vi "Create_Run_Dir.vi"(11 "Run":string) -> (0 "Run exists":bool, 1 "Time exists":bool, 2 "Date exists":bool, 3 "dup path":path)   [LabVIEW 2018]
panel:
  out "time string":string
  out "date string":string
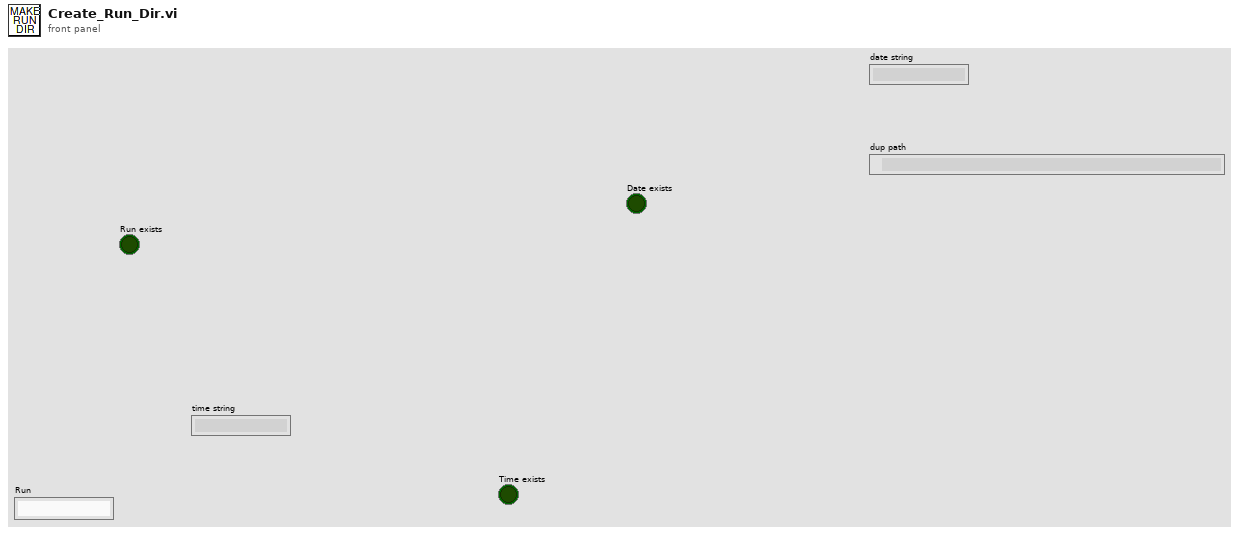
[diagram p1: front panel]
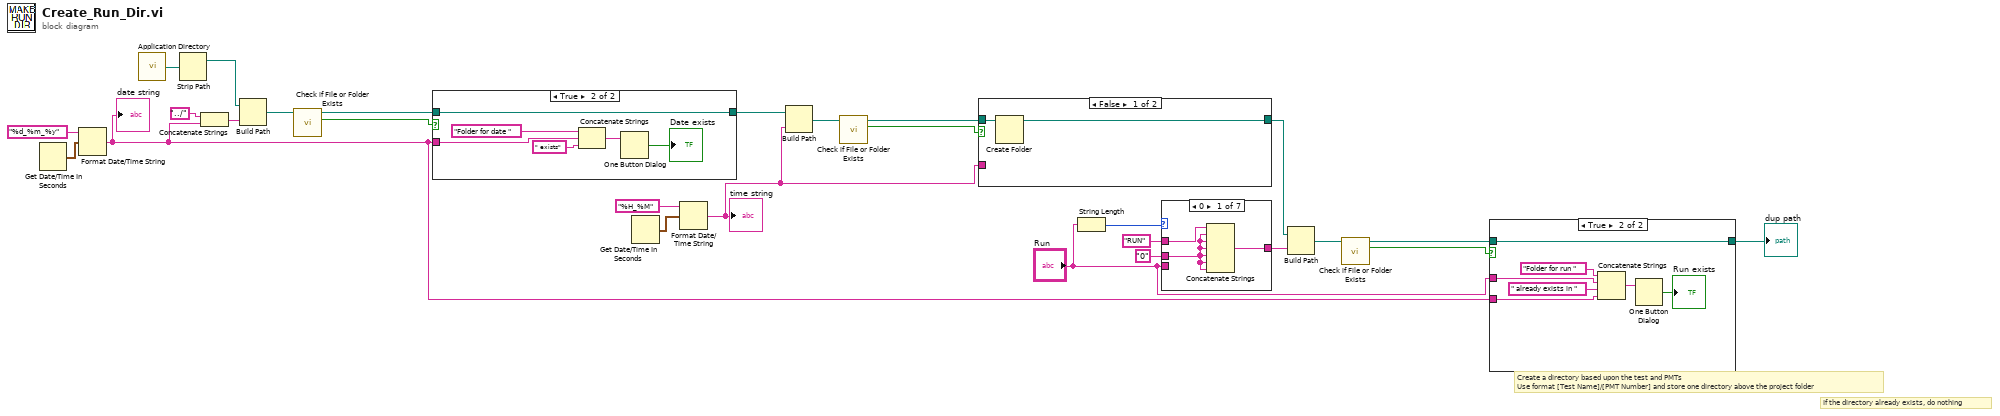
[diagram p0: block diagram]
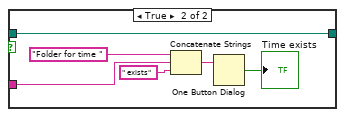
[diagram p2: hidden frame]
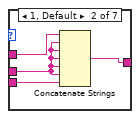
[diagram p3: hidden frame]
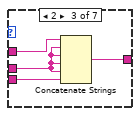
[diagram p4: hidden frame]
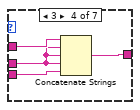
[diagram p5: hidden frame]
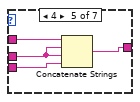
[diagram p6: hidden frame]
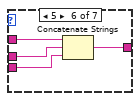
[diagram p7: hidden frame]
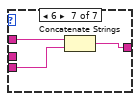
[diagram p8: hidden frame]
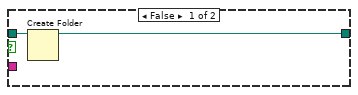
[diagram p9: hidden frame]
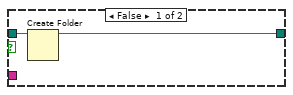
[diagram p10: hidden frame]
diagram:
  # "If the directory already exists, do nothing"
  # "Create a directory based upon the test and PMTs\nUse format [Test Name]/[PMT Number] and store one directory above the project folder"
  n1 = Get Date/Time In Seconds() -> (seconds since 1Jan1904=w22:timestamp)
  n2 = Format Date/Time String(time format string (%c)="%d_%m_%y", seconds (now)=w22) -> (date/time string=w11:string)  [unwired: 1 in]
  "date string" <- w11
  n3 = call <vilib>:"Application Directory.vi"() -> ("Application Directory"=w27:path)
  n4 = Strip Path(path=w27) -> (stripped path=w20:path)  [unwired: 1 out]
  n5 = Concatenate Strings("../" ("string"), w11) -> (w9:string)
  n6 = Build Path(base path=w20, name or relative path=w9) -> (appended path=w18:path)
  n7 = call <vilib>:"Check if File or Folder Exists.vi"("path"=w18) -> ("file or folder exists?"=w19:bool, "dup path"=w17:path)  [unwired: 8 in, 1 out]
  n8 = case shown="True" w19 {
    tunnel: w17 -> [w29 w35]
    tunnel: [w28 w35] -> w3
    tunnel: w11 -> [_ w31]
    frame False {
      n9 = Create Folder(path (use dialog)=w29) -> (created path=w28:path)  [unwired: 2 in, 2 out]
    }
    frame True {
      n10 = Concatenate Strings("Folder for date " ("message"), w31, " exists" ("string")) -> (w33:string)
      n11 = One Button Dialog(message=w33) -> (true=→"Date exists":bool)  [unwired: 1 in]
    }
  }
  n12 = Get Date/Time In Seconds() -> (seconds since 1Jan1904=w8:timestamp)
  n13 = Format Date/Time String(time format string (%c)="%H_%M", seconds (now)=w8) -> (date/time string=w1:string)  [unwired: 1 in]
  "time string" <- w1
  n14 = Build Path(base path=w3, name or relative path=w1) -> (appended path=w2:path)
  n15 = call <vilib>:"Check if File or Folder Exists.vi"("path"=w2) -> ("file or folder exists?"=w4:bool, "dup path"=w5:path)  [unwired: 8 in, 1 out]
  n16 = case shown="False" w4 {
    tunnel: w5 -> [w37 w43]
    tunnel: [w36 w43] -> w6
    tunnel: w1 -> [_ w39]
    frame False {
      n17 = Create Folder(path (use dialog)=w37) -> (created path=w36:path)  [unwired: 2 in, 2 out]
    }
    frame True {
      n18 = Concatenate Strings("Folder for time " ("message"), w39, " exists" ("string")) -> (w41:string)
      n19 = One Button Dialog(message=w41) -> (true=→"Time exists":bool)  [unwired: 1 in]
    }
  }
  n20 = String Length(string="Run") -> (length=w16:i32)
  n21 = case shown="0" w16 {
    tunnel: "RUN" ("string") -> [w46 w50 w53 w58 w61 w65 w68]
    tunnel: [w44 w49 w54 w55 w62 w66 w69] -> w14
    tunnel: "Run" -> [_ w48 w51 w56 w59 w63 w67]
    tunnel: "0" ("string") -> [w45 w47 w52 w57 w60 w64 _]
    frame 0 {
      n22 = Concatenate Strings(w46, w45, w45, w45, w45, w45, w45) -> (w44:string)
    }
    frame 1, Default {
      n23 = Concatenate Strings(w50, w47, w47, w47, w47, w47, w48) -> (w49:string)
    }
    frame 2 {
      n24 = Concatenate Strings(w53, w52, w52, w52, w52, w51) -> (w54:string)
    }
    frame 3 {
      n25 = Concatenate Strings(w58, w57, w57, w57, w56) -> (w55:string)
    }
    frame 4 {
      n26 = Concatenate Strings(w61, w60, w60, w59) -> (w62:string)
    }
    frame 5 {
      n27 = Concatenate Strings(w65, w64, w63) -> (w66:string)
    }
    frame 6 {
      n28 = Concatenate Strings(w68, w67) -> (w69:string)
    }
  }
  n29 = Build Path(base path=w6, name or relative path=w14) -> (appended path=w23:path)
  n30 = call <vilib>:"Check if File or Folder Exists.vi"("path"=w23) -> ("file or folder exists?"=w26:bool, "dup path"=w25:path)  [unwired: 8 in, 1 out]
  n31 = case shown="True" w26 {
    tunnel: w25 -> [w71 w78]
    tunnel: [w70 w78] -> w24
    tunnel: "Run" -> [_ w73]
    tunnel: w11 -> [_ w72]
    frame False {
      n32 = Create Folder(path (use dialog)=w71) -> (created path=w70:path)  [unwired: 2 in, 2 out]
    }
    frame True {
      n33 = Concatenate Strings("Folder for run " ("message"), w73, " already exists in " ("string"), w72) -> (w77:string)
      n34 = One Button Dialog(message=w77) -> (true=→"Run exists":bool)  [unwired: 1 in]
    }
  }
  "dup path" <- w24
